vi "SerialGlobals.vi"() -> ()   [LabVIEW 2010]
panel:
  in  "VISA resource name":refnum<visa-resource-name>="COM1"
  in  "Baud rate":u32=115200
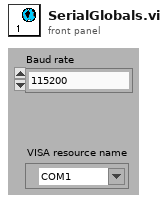
[diagram p1: front panel]
diagram:
